vi "Untitled 1.vi"() -> ()   [LabVIEW 2015]
uses:
  <vilib>/ptbypt/NI_PtbyPt.lvlib
panel:
  out "Waveform Chart 3":dynamicdata(graph) caption="Waveform Chart 2"
  out "Waveform Chart 2":dynamicdata(graph)
  in  "stop":bool
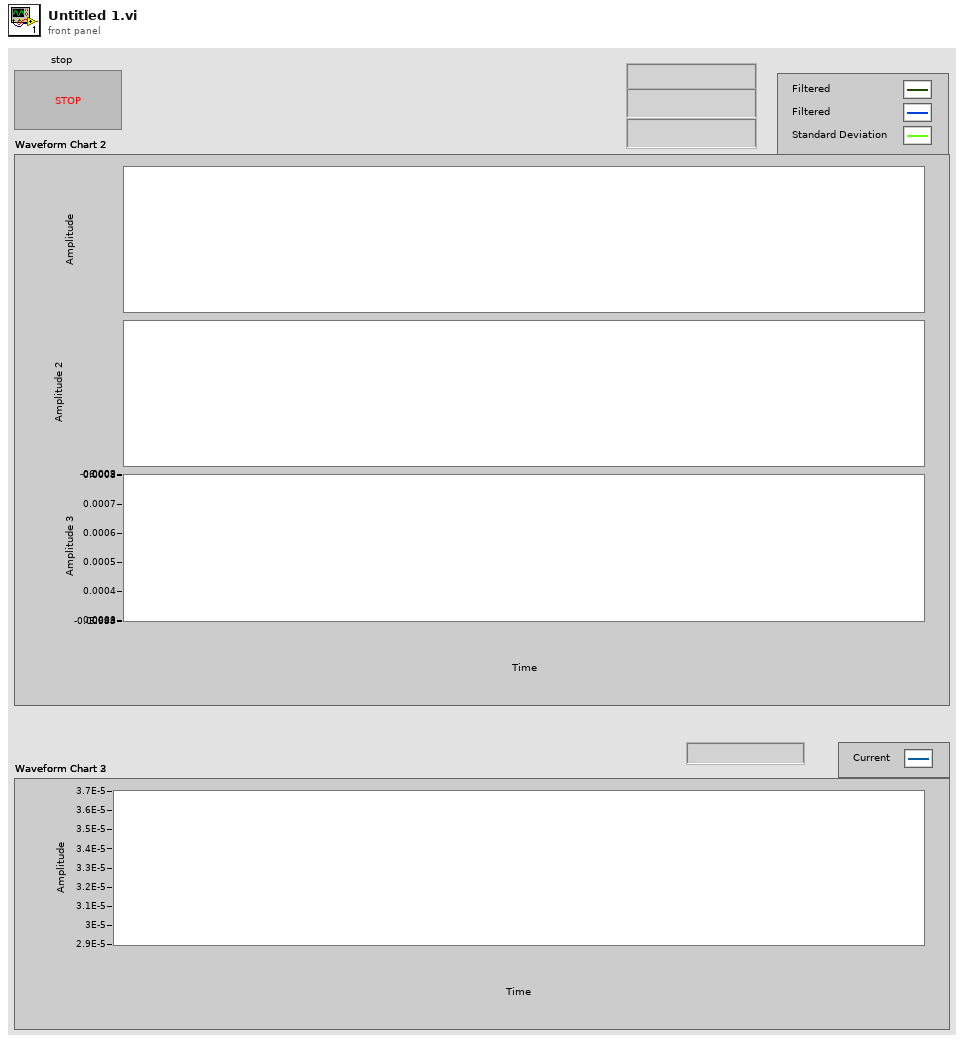
[diagram p1: front panel]
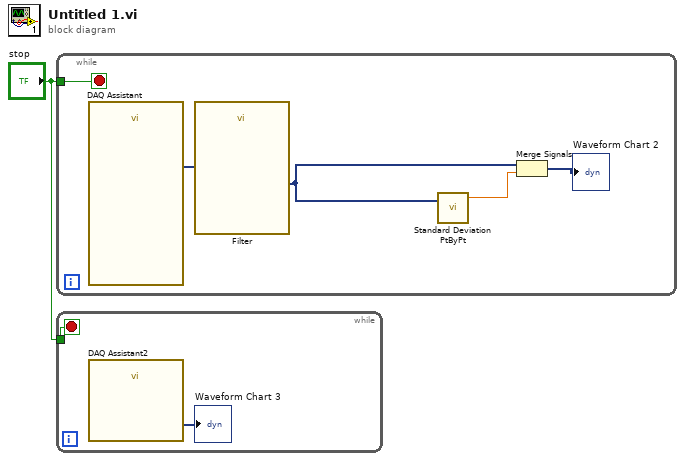
[diagram p0: block diagram]
diagram:
  n1 = while {
    tunnel: "stop" -> [w5]
    stop <- w5 stop-if-true
    n2 = call "DAQ Assistant"() -> ("data"=w6:dynamicdata)  [unwired: 17 in, 2 out]
    n3 = call "Filter"("Signal"=w6) -> ("Filtered Signal"=w3:dynamicdata)  [unwired: 9 in, 1 out]
    n4 = call <vilib>:"Standard Deviation PtByPt.vi"("x"=w3) -> ("standard deviation"=w4:dbl)  [unwired: 2 in, 2 out]
    n5 = Merge Signals(w3, w4) -> (→"Waveform Chart 2":dynamicdata)
  }
  n6 = while {
    tunnel: "stop" -> [w8]
    stop <- w8 stop-if-true
    n7 = call "DAQ Assistant2"() -> ("data"=→"Waveform Chart 3":dynamicdata)  [unwired: 17 in, 2 out]
  }
